vi "Scan Registry for USB Device_LV2012_NI Verified.vi"() -> ()   [LabVIEW 2018]
doc: "This VI monitors the connection to any USB device, be that a flash memory stick, a keyboard, a web camera,etc.. using Windows Registry"
uses:
  <vilib>/registry/registry.llb/Registry RtKey.ctl
  <vilib>/registry/registry.llb/Registry SAM.ctl
  <vilib>/regexp/Match Regular Expression.xnode
panel:
  in  "error in (no error)":errorcluster
  out "error out":errorcluster
  in  "Device ID to Check if Present":string="051939001D4A1B03"
  out "Device Present?":bool
  # "Overview: This VI monitors the connection to any USB device, be that a flash memory stick, a keyboard, a web camera,etc.. using Windows Registry\nRequirements: LabVIEW 2012 (or compatible)\nInstructions:\n1. Plug a USB device into the system.\n2.  Open Windows Device Manager and locate the USB device.\n3. Under the details tab Note down the device instance ID, this varies from device to device but the last part after the last \"\\\" is usually sufficient.\n4. Or Open the windows registry (type \"regedit\" in the run menu).\n5. Navigate to HKEY_LOCAL_MACHINE\\SYSTEM\\CurrentControlSet\\services.\n6. Locate the device ID in one of the USB registry keys ( device must be connected,  might be easier to search for it).\n7. Note down the subkey (folder) the device is stored in.  By default the VI uses USBSTOR, usbccgp, usbehci, usbaudio.\n8. If the device falls under one of these subkeys you are ready to go.  If not add the sub key to the paths in the VI.\n9. Enter the device ID in the Device ID Control (similar to the default value of the control)\n10.Run the VI"
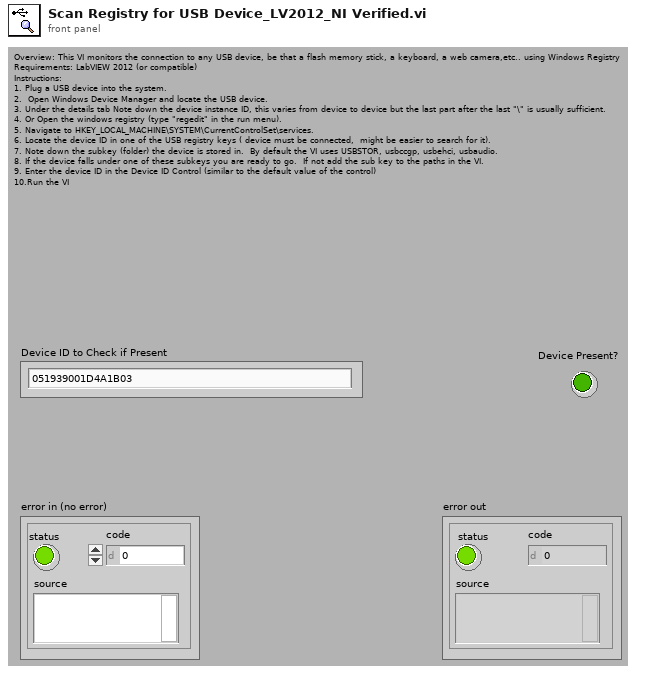
[diagram p1: front panel]
types:
  T1 = typedef "Registry RtKey.ctl" = enum32{"HKEY_CLASSES_ROOT", "HKEY_CURRENT_USER", "HKEY_LOCAL_MACHINE", "HKEY_USERS", "HKEY_PERFORMANCE_DATA", "HKEY_CURRENT_CONFIG", "HKEY_DYN_DATA"}
  T2 = typedef "Registry SAM.ctl" = enum32{"KEY_QUERY_VALUE", "KEY_SET_VALUE", "KEY_CREATE_SUB_KEY", "KEY_ENUMERATE_SUB_KEYS", "KEY_NOTIFY", "KEY_CREATE_LINK", "KEY_READ", "KEY_WRITE", "KEY_ALL_ACCESS", "KEY_READ | KEY_WRITE"}
  T3 = typedef "Registry refnum.ctl" = refnum<k1>
  T4 = cluster{"numValues":i32, "maxValueNameLen":i32, "maxValueDataLen":i32}
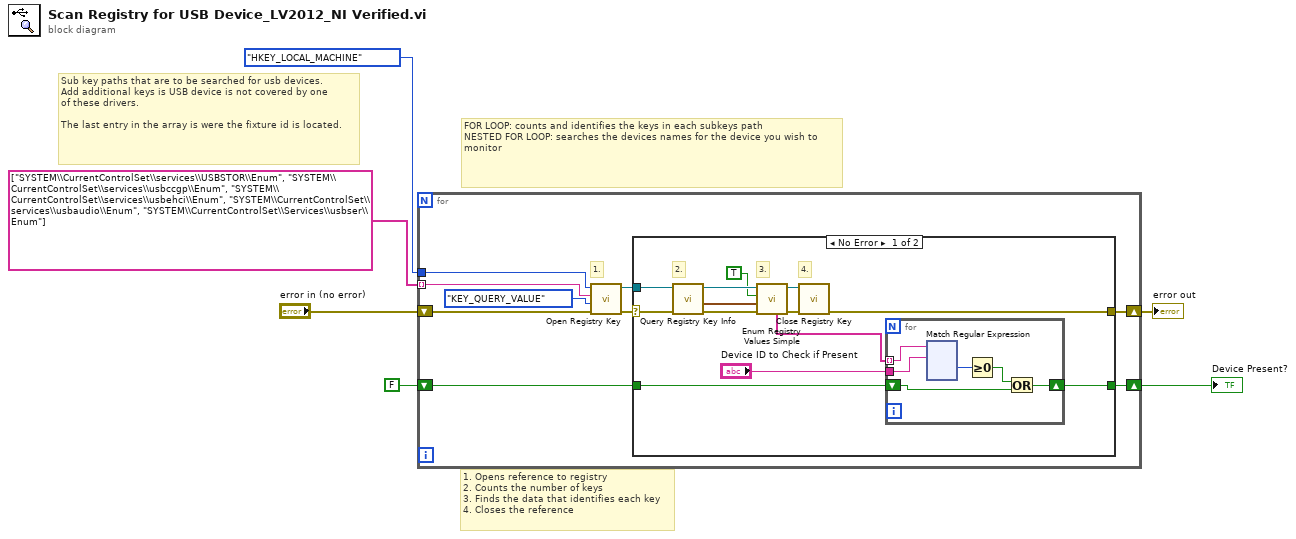
[diagram p0: block diagram]
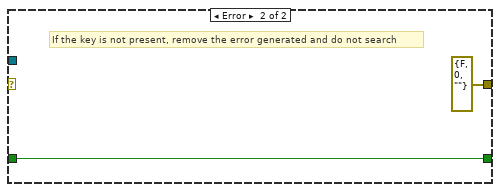
[diagram p2: hidden frame]
diagram:
  # "1. Opens reference to registry\n2. Counts the number of keys\n3. Finds the data that identifies each key\n4. Closes the reference"
  # "FOR LOOP: counts and identifies the keys in each subkeys path\nNESTED FOR LOOP: searches the devices names for the device you wish to monitor"
  # "Sub key paths that are to be searched for usb devices.\nAdd additional keys is USB device is not covered by one\nof these drivers.\n\nThe last entry in the array is were the fixture id is located."
  n1 = for {
    tunnel: string[] ["SYSTEM\\CurrentControlSet\\services\\USBSTOR\\Enum", "SYSTEM\\CurrentControlSet\\services\\usbccgp\\Enum", "SYSTEM\\CurrentControlSet\\services\\usbehci\\Enum", "SYSTEM\\CurrentControlSet\\services\\usbaudio\\Enum", "SYSTEM\\CurrentControlSet\\Services\\usbser\\Enum"] -> [w15] mode=indexing
    shift-right: [w11] -> w5
    shift-left: "error in (no error)" -> [w12]
    shift-right: [w9] -> w3
    shift-left: FALSE -> [w10]
    tunnel: Registry_RtKey."HKEY_LOCAL_MACHINE" ("root key (HKEY_LOCAL_MACHINE)") -> [w8]
    # "1."
    n2 = call <vilib>:"Open Registry Key.vi"("error in (no error)"=w12, "security access mask (KEY_READ | KEY_WRITE)"=Registry_SAM."KEY_QUERY_VALUE", "subkey"=w15, "root key (HKEY_LOCAL_MACHINE)"=w8) -> ("error out"=w14:errorcluster, "refnum out"=w13:T3)  [unwired: 6 out]
    n3 = case shown="No Error" w14 {
      selector: w14 -> [w19 _]
      tunnel: w13 -> [w20 _]
      tunnel: [w18 errorcluster {"status"=FALSE, "code"=0, "source"=""} ("error in (no error)")] -> w11
      tunnel: w10 -> [w17 w146]
      tunnel: [w16 w146] -> w9
      frame No Error {
        # "4."
        # "3."
        # "2."
        n4 = call <vilib>:"Query Registry Key Info.vi"("error in (no error)"=w19, "refnum"=w20) -> ("error out"=w28:errorcluster, "value info"=w21:T4, "refnum out"=w27:T3)  [unwired: 7 out]
        n5 = call <vilib>:"Enum Registry Values Simple.vi"("error in (no error)"=w28, "value info"=w21, "retrieve data? (F)"=TRUE, "refnum"=w27) -> ("error out"=w23:errorcluster, "refnum out"=w22:T3, "String/Binary data"=w24:string[])  [unwired: 5 out]
        n6 = call <vilib>:"Close Registry Key.vi"("error in (no error)"=w23, "refnum"=w22) -> ("error out"=w18:errorcluster)  [unwired: 5 out]
        n7 = for {
          tunnel: "Device ID to Check if Present" -> [w34]
          tunnel: w24 -> [w33] mode=indexing
          shift-right: [w29] -> w16
          shift-left: w17 -> [w32]
          n8 = xnode "Match Regular Expression"("input string"=w33, "regular expression"=w34) -> ("offset past match"=w31:i32)  [unwired: 3 in, 5 out]
          n9 = Greater Or Equal To 0?(x=w31) -> (x >= 0?=w30:bool)
          n10 = Or(x=w30, y=w32) -> (x .or. y?=w29:bool)
        }
      }
      frame Error {
        # "If the key is not present, remove the error generated and do not search"
      }
    }
  }
  "error out" <- w5
  "Device Present?" <- w3
